vi "rev_throttle.vi"() -> (3 "t PWM":dbl=-2.0)   [LabVIEW 2015]
uses:
  RIOGlobal.vi
panel:
  in  "kd":dbl=1.0
  in  "y":dbl=1.0
  in  "Boolean":bool
  in  "dead zone":dbl
  in  "friction":dbl=500.0
  in  "kp":dbl=20.0
  in  "ki":dbl=2.0
  in  "gm":dbl=0.01
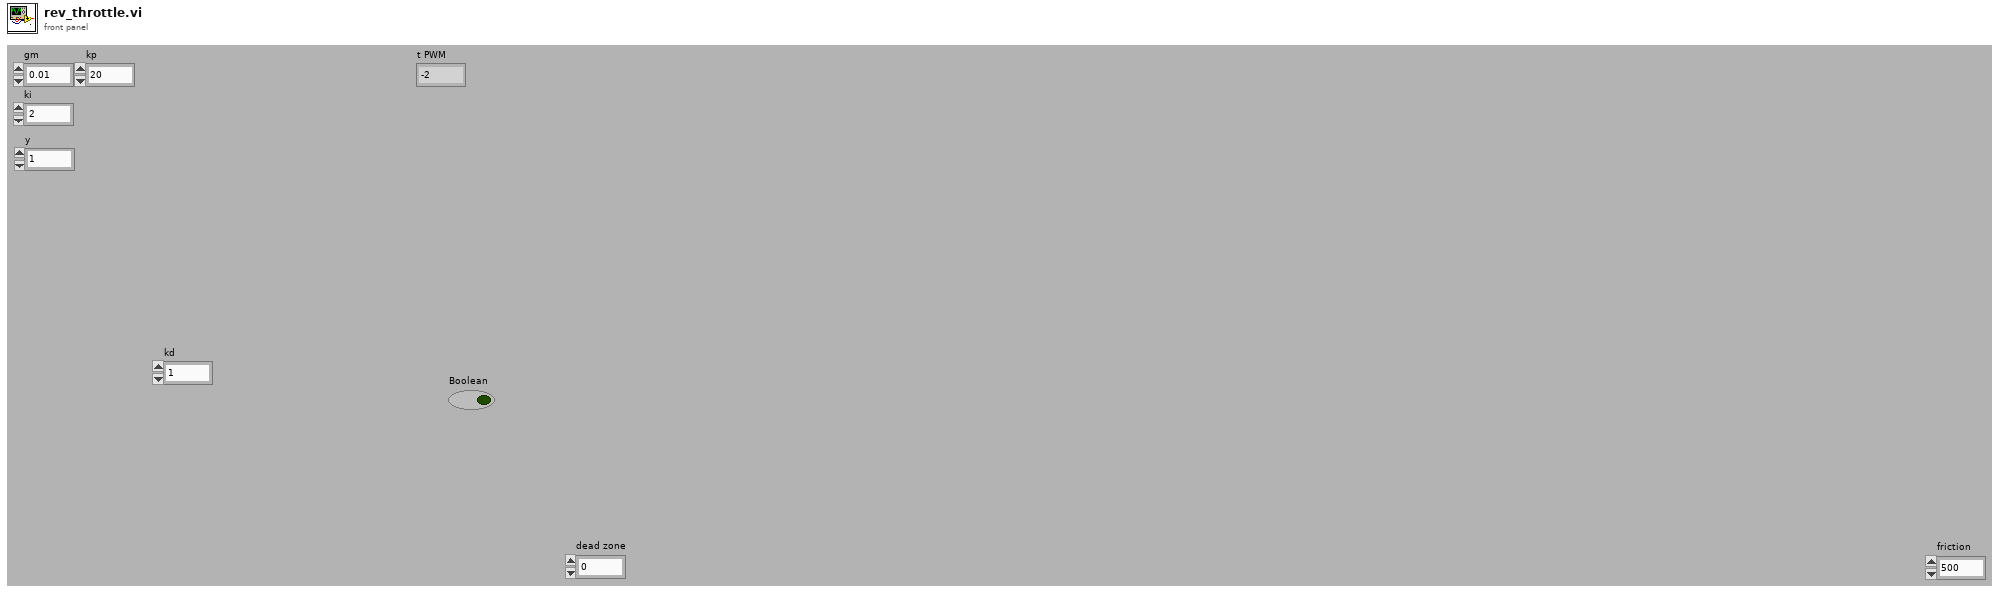
[diagram p1: front panel]
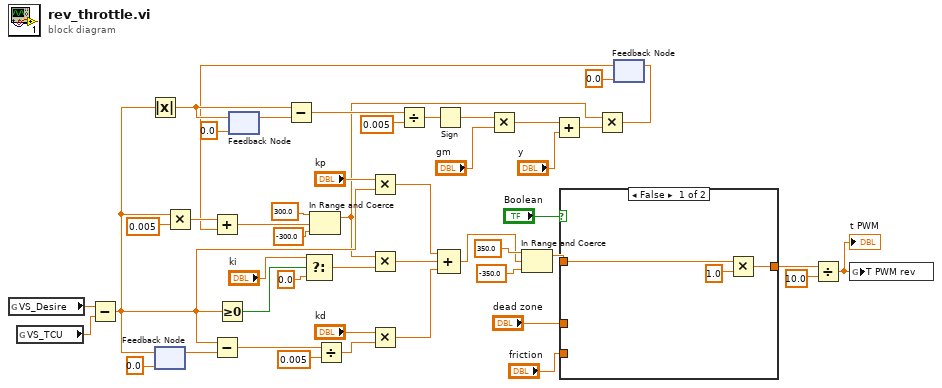
[diagram p0: block diagram]
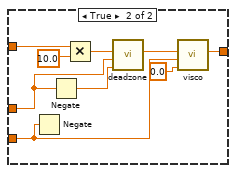
[diagram p2: hidden frame]
diagram:
  n1 = global read "RIOGlobal.vi" "VS_Desire"() -> (w47:dbl)
  n2 = global read "RIOGlobal.vi" "VS_TCU"() -> (w46:dbl)
  n3 = Subtract(x=w47, y=w46) -> (x-y=w13:dbl)
  n4 = Absolute Value(x=w13) -> (abs(x)=w44:dbl)
  n5 = feedback #1(0.0) -> (w14:dbl)
  n6 = feedback-in #1(w13) -> ()
  n7 = Multiply(x=w13, y=0.005) -> (x*y=w33:dbl)
  n8 = Subtract(x=w13, y=w14) -> (x-y=w15:dbl)
  n9 = Greater Or Equal To 0?(x=w13) -> (x >= 0?=w21:bool)
  n10 = feedback #2(0.0) -> (w43:dbl)
  n11 = feedback-in #2(w44) -> ()
  n12 = Subtract(x=w44, y=w43) -> (x-y=w42:dbl)
  n13 = Select(t="ki", s=w21, f=0.0) -> (s? t:f=w18:dbl)
  n14 = Divide(x=w15, y=0.005) -> (x/y=w11:dbl)
  n15 = Multiply(x="kp", y=w13) -> (x*y=w30:dbl)
  n16 = Multiply(x="kd", y=w11) -> (x*y=w10:dbl)
  n17 = Divide(x=w42, y=0.005) -> (x/y=w40:dbl)
  n18 = Sign(1:w40) -> (0:w39:dbl)
  n19 = Multiply(x=w39, y="gm") -> (x*y=w37:dbl)
  n20 = Add(x=w37, y="y") -> (x+y=w35:dbl)
  n21 = feedback #3(0.0) -> (w32:dbl)
  n22 = Add(x=w33, y=w32) -> (x+y=w1:dbl)
  n23 = In Range and Coerce(upper limit=300.0 ("max"), x=w1, lower limit=-300.0 ("min")) -> (coerced(x)=w4:dbl)  [unwired: 1 out]
  n24 = Multiply(x=w4, y=w18) -> (x*y=w29:dbl)
  n25 = Compound Arithmetic op=ADD(w30, w29, w10) -> (w6:dbl)
  n26 = In Range and Coerce(upper limit=350.0 ("max"), x=w6, lower limit=-350.0 ("min")) -> (coerced(x)=w5:dbl)  [unwired: 1 out]
  n27 = case shown="False" "Boolean" {
    tunnel: [w48 w58] -> w23
    tunnel: "friction" -> [_ w57]
    tunnel: "dead zone" -> [_ w54]
    tunnel: w5 -> [w49 w53]
    frame False {
      n28 = Multiply(x=w49, y=1.0) -> (x*y=w48:dbl)
    }
    frame True {
      n29 = Negate(x=w57) -> ()  [unwired: 1 out]
      n30 = Negate(x=w54) -> (-x=w52:dbl)
      n31 = Multiply(x=w53, y=10.0) -> (x*y=w55:dbl)
      n32 = call "deadzone.vi"("min"=w52, "max"=w54, "x"=w55) -> ("dead zone"=w56:dbl)  [unwired: 8 in]
      n33 = call "visco.vi"("min"=0.0, "max"=w57, "input"=w56) -> ("output"=w58:dbl)  [unwired: 8 in]
    }
  }
  n34 = Multiply(x=w4, y=w35) -> (x*y=w34:dbl)
  n35 = feedback-in #3(w34) -> ()
  n36 = Divide(x=w23, y=10.0) -> (x/y=w9:dbl)
  "t PWM" <- w9
  n37 = global write "RIOGlobal.vi" "T PWM rev"(w9) -> ()
